vi "hcE_fortran.vi"(4 "nd":i32, 5 "ng":i32, 6 "ns":i32, 7 "n":i32, 9 "d":dbl[](array[numeric]), 10 "ic":i32[](array[numeric]), 11 "x (data)":dbl[](array[numeric])) -> (1 "d (out)":dbl[](array[numeric]), 2 "ic (out)":i32[](array[numeric]), 3 "x (data out)":dbl[](array[numeric]))   [LabVIEW 2014]
panel:
  out "iopt":i32
  out "jopt":i32
  out "iold":i32
  out "jold":i32
  out "dold":dbl
  out "dij":dbl
  out "jk":i32
  out "ik":i32
  out "ii":i32
  out "icj":i32
  out "ici":i32
  out "ij":i32
  out "dopt":dbl
  out "sij":dbl
  out "nj":i32
  out "rj":dbl
  out "sj":dbl
  out "si":dbl
  out "rij":dbl
  out "ri":dbl
  out "nij":i32
  out "ni":i32
  out "FLMAX":dbl=1.797693134862e+308
  out "k":i32
  out "m":i32
  out "j":i32
  out "i":i32
  out "Is":i32
  out "Io":i32
  out "II":i32
  out "Id":i32
  out "Ig":i32
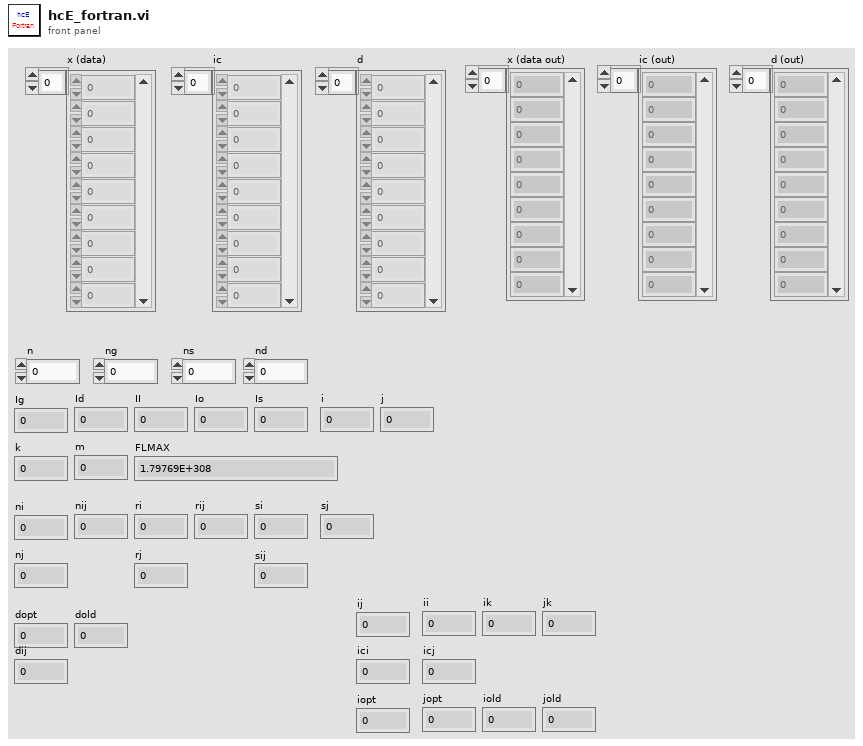
[diagram p1: front panel]
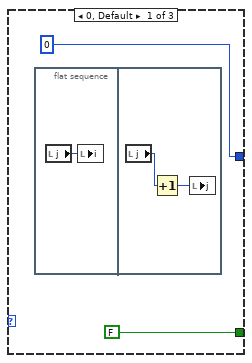
[diagram p2: hidden frame]
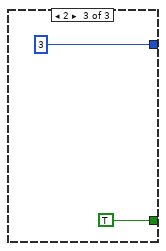
[diagram p3: hidden frame]
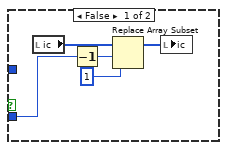
[diagram p6: hidden frame]
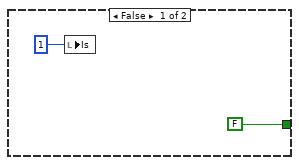
[diagram p8: hidden frame]
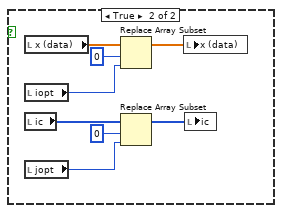
[diagram p9: hidden frame]
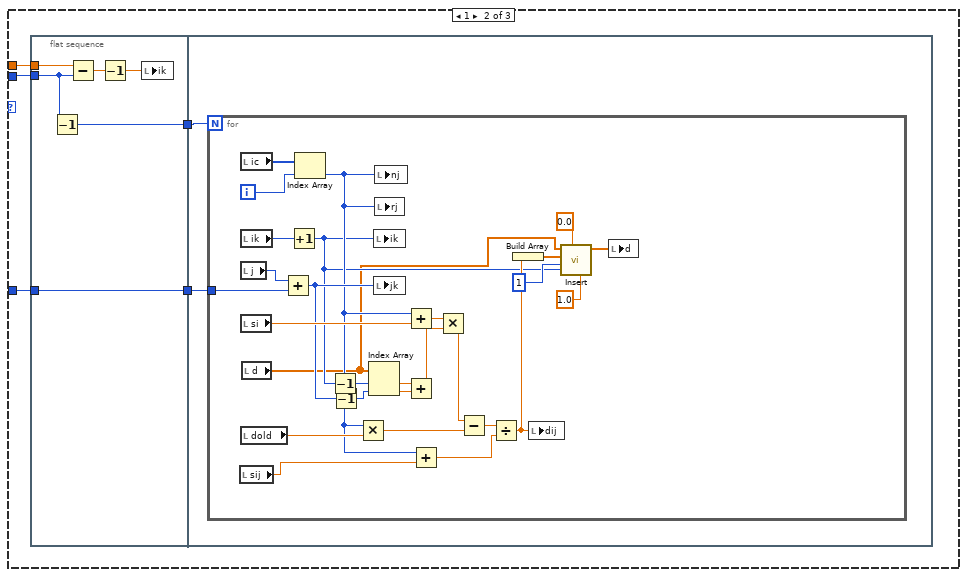
[diagram p12: hidden frame]
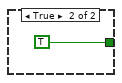
[diagram p13: hidden frame]
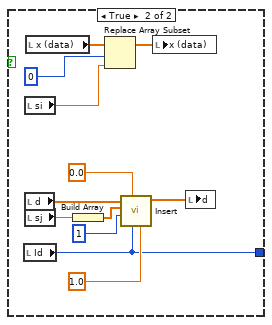
[diagram p14: hidden frame]
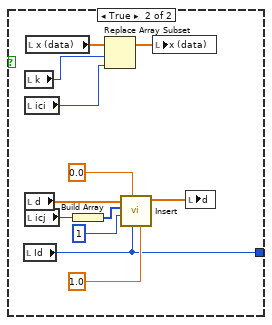
[diagram p16: hidden frame]
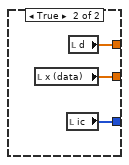
[diagram p17: hidden frame]
diagram:
  n1 = flat-sequence {
    tunnel: [w15] -> w5
    tunnel: w5 -> [w38]
    tunnel: [w37] -> w4
    tunnel: w4 -> [w188]
    tunnel: [w187] -> w2
    tunnel: [w186] -> w1
    tunnel: [w185] -> w3
    frame #0 {
      n2 = Decrement(x="ng") -> (x-1=w14:i32)
      n3 = Multiply(x="ng", y=w14) -> (x*y=w13:i32)
      n4 = Subtract(x="nd", y="ng") -> (x-y=→"II":i32)
      n5 = Divide(x=w13, y=2) -> (x/y=→"Id":dbl)
      "Ig" <- "ng"
      "Io" <- "nd"
      "i" <- 1 ("i")
      "j" <- 2 ("j")
    }
    frame #1 {
      # "i = 1\n      j = 2\n 1    continue\n        icj = ic(j)\n        if (icj .ne. j) goto 2\n        if (j .eq. lg)  goto 3\n        i = j\n        j = j + 1\n      goto 1"
      n6 = while {
        tunnel: [w17] -> w15
        i -> [w27]
        stop <- w18 stop-if-true
        # "j = 2\n(i or here is j)"
        n7 = local read "Ig"() -> (w23:i32)
        n8 = local read "ic"() -> (w26:i32[])
        n9 = Increment(x=w27) -> (x+1=w24:i32)
        n10 = Decrement(x=w24) -> (x-1=w16:i32)
        n11 = Index Array(array=w26, index=w16) -> (element=w25:i32)
        n12 = Equal?(x=w23, y=w24) -> (x = y?=w21:bool)
        n13 = Not Equal?(x=w24, y=w25) -> (x != y?=w22:bool)
        n14 = Build Array(w22, w21) -> (w20:bool[])
        n15 = call "Case_Selector.vi"("Array"=w20) -> ("Case Numer"=w19:i32)  [unwired: 10 in]
        n16 = case shown="1" w19 {
          tunnel: [FALSE TRUE TRUE] -> w18
          tunnel: [0 2 3] -> w17
          frame 0, Default {
            n17 = flat-sequence {
              frame #0 {
                n18 = local read "j"() -> (w30:i32)
                n19 = local write "i"(w30) -> ()
              }
              frame #1 {
                n20 = local read "j"() -> (w32:i32)
                n21 = Increment(x=w32) -> (x+1=w31:i32)
                n22 = local write "j"(w31) -> ()
              }
            }
          }
          frame 1 {
          }
          frame 2 {
          }
        }
      }
    }
    frame #2 {
      # "Fortran statement 2 and 3 part"
      n23 = flat-sequence {
        tunnel: w38 -> [w39]
        tunnel: [w68] -> w37
        frame #0 {
          # "Fortran statement 2"
          n24 = case shown="2, Default" w39 {
            frame 2, Default {
              n25 = flat-sequence {
                frame #0 {
                  n26 = local read "i"() -> (w42:i32)
                  n27 = local read "j"() -> (w40:i32)
                  n28 = Increment(x=w40) -> (x+1=w41:i32)
                  n29 = local write "k"(w42) -> ()
                  n30 = local write "m"(w41) -> ()
                }
                frame #1 {
                  n31 = while {
                    i -> [w52]
                    stop <- w49 stop-if-true
                    n32 = local read "ic"() -> (w47:i32[])
                    n33 = local read "k"() -> (w46:i32)
                    n34 = local read "m"() -> (w51:i32)
                    n35 = local read "n"() -> (w50:i32)
                    n36 = Add(x=w51, y=w52) -> (x+y=w48:i32)
                    n37 = Decrement(x=w48) -> (x-1=w44:i32)
                    n38 = Greater Or Equal?(x=w48, y=w50) -> (x >= y?=w49:bool)
                    n39 = local write "j"(w48) -> ()
                    n40 = Index Array(array=w47, index=w44) -> (element=w43:i32)
                    n41 = Greater?(x=w43, y=w46) -> (0:w45:bool)
                    n42 = case shown="True" w45 {
                      tunnel: w43 -> [_ w53]
                      frame False {
                      }
                      frame True {
                        n43 = flat-sequence {
                          tunnel: [w55] -> w54
                          tunnel: w53 -> [w55]
                          tunnel: w54 -> [w61]
                          frame #0 {
                            n44 = local read "k"() -> (w57:i32)
                            n45 = Increment(x=w57) -> (x+1=w56:i32)
                            n46 = local write "k"(w56) -> ()
                          }
                          frame #1 {
                            n47 = local read "x (data)"() -> (w67:dbl[])
                            n48 = local read "k"() -> (w64:i32)
                            n49 = local read "j"() -> (w63:i32)
                            n50 = local read "ic"() -> (w65:i32[])
                            n51 = Decrement(x=w64) -> (x-1=w60:i32)
                            n52 = call "swap.vi"("j"=w63, "k"=w64, "Array"=w67) -> ("Array (swap)"=w66:dbl[])  [unwired: 8 in]
                            n53 = Index Array(array=w65, index=w60) -> (element=w62:i32)
                            n54 = Decrement(x=w63) -> (x-1=w59:i32)
                            n55 = Replace Array Subset(array=w65, new element #1=w62, index #1=w59, new element #2=w61, index #2=w60) -> (w58:i32[])
                            n56 = local write "x (data)"(w66) -> ()
                            n57 = local write "ic"(w58) -> ()
                          }
                        }
                      }
                    }
                  }
                }
              }
            }
            frame 3 {
            }
          }
        }
        frame #1 {
          # "Fortran statement 3"
          n58 = flat-sequence {
            tunnel: [w156] -> w68
            frame #0 {
              n59 = while {
                i -> [w72]
                stop <- w74 stop-if-true
                n60 = local read "ic"() -> (w73:i32[])
                n61 = local read "n"() -> (w75:i32)
                n62 = Increment(x=w72) -> (x+1=w70:i32)
                n63 = Index Array(array=w73, index=w72) -> (element=w69:i32)
                n64 = Greater Or Equal?(x=w70, y=w75) -> (x >= y?=w74:bool)
                n65 = local write "i"(w69) -> ()
                n66 = local write "j"(w70) -> ()
                n67 = Not Equal?(x=w69, y=w70) -> (x != y?=w71:bool)
                n68 = case shown="True" w71 {
                  tunnel: w70 -> [w79 w82]
                  tunnel: w69 -> [_ w81]
                  frame False {
                    n69 = local read "ic"() -> (w80:i32[])
                    n70 = Decrement(x=w79) -> (x-1=w78:i32)
                    n71 = Replace Array Subset(array=w80, new element=1 ("new element/subarray"), index=w78) -> (w76:i32[])
                    n72 = local write "ic"(w76) -> ()
                  }
                  frame True {
                    n73 = flat-sequence {
                      tunnel: w82 -> [w91]
                      tunnel: w81 -> [w87]
                      frame #0 {
                        n74 = Decrement(x=w87) -> (x-1=w85:i32)
                        n75 = local read "ic"() -> (w88:i32[])
                        n76 = Decrement(x=w91) -> (x-1=w90:i32)
                        n77 = Index Array(array=w88, index=w85) -> (element=w86:i32)
                        n78 = Increment(x=w86) -> (x+1=w84:i32)
                        n79 = local write "nij"(w84) -> ()
                        n80 = local write "ni"(w86) -> ()
                        n81 = Replace Array Subset(array=w88, new element #1=0 ("new element/subarray"), index #1=w90, new element #2=w84, index #2=w85) -> (w83:i32[])
                        n82 = local write "ic"(w83) -> ()
                      }
                      frame #1 {
                        n83 = local read "nij"() -> (w107:i32)
                        n84 = local read "ni"() -> (w105:i32)
                        n85 = local read "x (data)"() -> (w96:dbl[])
                        n86 = local read "i"() -> (w104:i32)
                        n87 = local read "j"() -> (w103:i32)
                        n88 = Decrement(x=w103) -> (x-1=w95:i32)
                        n89 = Decrement(x=w104) -> (x-1=w94:i32)
                        n90 = Divide(x=1.0, y=w107) -> (x/y=w106:dbl)
                        n91 = Index Array(array=w96, index #1=w94, index #2=w95) -> (element #1=w102:dbl, element #2=w101:dbl)
                        n92 = Square Root(x=w106) -> (sqrt(x)=w99:dbl)
                        n93 = Multiply(x=w99, y=w105) -> (x*y=w100:dbl)
                        n94 = Multiply(x=w102, y=w100) -> (x*y=w98:dbl)
                        n95 = Multiply(x=w101, y=w99) -> (x*y=w97:dbl)
                        n96 = local write "rij"(w107) -> ()
                        n97 = local write "sj"(w99) -> ()
                        n98 = local write "si"(w100) -> ()
                        n99 = local write "ri"(w105) -> ()
                        n100 = Add(x=w98, y=w97) -> (x+y=w93:dbl)
                        n101 = Replace Array Subset(array=w96, new element=w93, index=w94) -> (w92:dbl[])
                        n102 = local write "x (data)"(w92) -> ()
                      }
                    }
                  }
                }
              }
            }
            frame #1 {
              n103 = local read "FLMAX"() -> (w110:dbl)
              n104 = local write "dopt"(w110) -> ()
              n105 = local write "ij"(0 ("ij")) -> ()
            }
            frame #2 {
              n106 = while {
                i -> [w115]
                stop <- w112 stop-if-true
                n107 = local read "Ig"() -> (w113:i32)
                n108 = flat-sequence {
                  tunnel: w111 -> [w119]
                  frame #0 {
                    n109 = local read "ic"() -> (w118:i32[])
                    n110 = Decrement(x=w119) -> (x-1=w117:i32)
                    n111 = local write "j"(w119) -> ()
                    n112 = Index Array(array=w118, index=w117) -> (element=w116:i32)
                    n113 = local write "rij"(w116) -> ()
                    n114 = local write "nj"(w116) -> ()
                  }
                  frame #1 {
                    n115 = while {
                      i -> [w141]
                      stop <- w150 stop-if-true
                      # "x(i), x(j)"
                      # "ic(i)"
                      n116 = local read "ic"() -> (w149:i32[])
                      n117 = local read "j"() -> (w152:i32)
                      n118 = Increment(x=w141) -> (x+1=w120:i32)
                      n119 = Decrement(x=w152) -> (x-1=w151:i32)
                      n120 = Index Array(array=w149, index=w141) -> (element=w147:i32)
                      n121 = local read "nj"() -> (w148:i32)
                      n122 = local read "rij"() -> (w143:dbl)
                      n123 = local read "x (data)"() -> (w142:dbl[])
                      n124 = local read "j"() -> (w140:i32)
                      n125 = local read "dopt"() -> (w122:dbl)
                      n126 = local read "d"() -> (w129:dbl[])
                      n127 = local read "ij"() -> (w131:i32)
                      n128 = Greater Or Equal?(x=w120, y=w151) -> (x >= y?=w150:bool)
                      n129 = Decrement(x=w140) -> (x-1=w139:i32)
                      n130 = Increment(x=w131) -> (x+1=w126:i32)
                      n131 = local write "i"(w120) -> ()
                      n132 = Add(x=w147, y=w148) -> (x+y=w144:i32)
                      n133 = Divide(x=w147, y=w144) -> (x/y=w145:dbl)
                      n134 = Divide(x=w143, y=w144) -> (x/y=w146:dbl)
                      n135 = Index Array(array=w142, index #1=w141, index #2=w139) -> (element #1=w138:dbl, element #2=w136:dbl)
                      n136 = Square Root(x=w145) -> (sqrt(x)=w135:dbl)
                      n137 = Square Root(x=w146) -> (sqrt(x)=w137:dbl)
                      n138 = Multiply(x=w138, y=w137) -> (x*y=w134:dbl)
                      n139 = Multiply(x=w136, y=w135) -> (x*y=w133:dbl)
                      n140 = Subtract(x=w134, y=w133) -> (x-y=w132:dbl)
                      n141 = Square(x=w132) -> (x^2=w121:dbl)
                      n142 = Less Or Equal?(x=w121, y=w122) -> (x <= y?=w123:bool)
                      n143 = case shown="True" w123 {
                        tunnel: w121 -> [_ w155]
                        tunnel: w120 -> [_ w154]
                        frame False {
                        }
                        frame True {
                          n144 = local read "j"() -> (w153:i32)
                          n145 = local write "dopt"(w155) -> ()
                          n146 = local write "iopt"(w154) -> ()
                          n147 = local write "jopt"(w153) -> ()
                        }
                      }
                      n148 = Build Array(w121) -> (w124:dbl[])
                      n149 = call "Insert.vi"("da"=1.0, "iy"=w126, "dy weight"=0.0, "ix"=1 ("iy"), "dx"=w124, "dy in"=w129) -> ("dy out"=w128:dbl[])  [unwired: 5 in]
                      n150 = local write "dij"(w121) -> ()
                      n151 = local write "ni"(w147) -> ()
                      n152 = local write "ri"(w147) -> ()
                      n153 = local write "nij"(w144) -> ()
                      n154 = local write "rij"(w144) -> ()
                      n155 = local write "si"(w135) -> ()
                      n156 = local write "sj"(w137) -> ()
                      n157 = local write "d"(w128) -> ()
                      n158 = local write "ij"(w126) -> ()
                    }
                  }
                }
                n159 = Add(x=w115, y=2) -> (x+y=w111:i32)
                n160 = Greater Or Equal?(x=w111, y=w113) -> (x >= y?=w112:bool)
              }
            }
            frame #3 {
              n161 = local read "ns"() -> (w159:i32)
              n162 = Equal?(x=w159, y=1) -> (x = y?=w157:bool)
              n163 = case shown="True" w157 {
                tunnel: [FALSE TRUE] -> w156
                frame False {
                  n164 = local write "Is"(1 ("Is")) -> ()
                }
                frame True {
                  n165 = local read "d"() -> (w167:dbl[])
                  n166 = local read "iopt"() -> (w164:i32)
                  n167 = local read "jopt"() -> (w163:i32)
                  n168 = Less?(x=w164, y=w163) -> (x < y?=w162:bool)
                  n169 = Index Array(array=w167, index=0) -> (element=w165:dbl)
                  n170 = case shown="False" w162 {
                    frame False {
                      n171 = local read "x (data)"() -> (w176:dbl[])
                      n172 = local read "jopt"() -> (w174:i32)
                      n173 = local read "ic"() -> (w170:i32[])
                      n174 = local read "iopt"() -> (w172:i32)
                      n175 = Replace Array Subset(array=w176, new element=w174, index=0) -> (w173:dbl[])
                      n176 = Replace Array Subset(array=w170, new element=w172, index=0) -> (w169:i32[])
                      n177 = local write "x (data)"(w173) -> ()
                      n178 = local write "ic"(w169) -> ()
                    }
                    frame True {
                      n179 = local read "x (data)"() -> (w184:dbl[])
                      n180 = local read "iopt"() -> (w182:i32)
                      n181 = local read "ic"() -> (w178:i32[])
                      n182 = local read "jopt"() -> (w180:i32)
                      n183 = Replace Array Subset(array=w184, new element=w182, index=0) -> (w181:dbl[])
                      n184 = Replace Array Subset(array=w178, new element=w180, index=0) -> (w177:i32[])
                      n185 = local write "x (data)"(w181) -> ()
                      n186 = local write "ic"(w177) -> ()
                    }
                  }
                  n187 = local write "dopt"(w165) -> ()
                }
              }
            }
          }
        }
      }
    }
    frame #3 {
      # "Fortran statement 100 and 300 part\nif ns == 1 than it should pass this part and return \n\n ****************************************************\n\n<prior parts...>\nif (ns .eq. 1) then\n        if (iopt .lt. jopt) then\n          x(1)  = dble(iopt)\n          ic(1) = jopt\n        else\n          x(1)  = dble(jopt)\n          ic(1) = iopt\n        end if\n        d(1)    = dopt\n        return\n      end if"
      n188 = case shown="False" w188 {
        tunnel: [w191 w527] -> w187
        tunnel: [w189 w526] -> w186
        tunnel: [w190 w525] -> w185
        frame False {
          n189 = flat-sequence {
            tunnel: [w351] -> w191
            tunnel: [w350] -> w190
            tunnel: [w349] -> w189
            frame #0 {
              # "Fortran statement 100"
              n190 = while {
                stop <- w192 stop-if-true
                n191 = flat-sequence {
                  tunnel: [w342] -> w192
                  frame #0 {
                    n192 = local read "ic"() -> (w200:i32[])
                    n193 = local read "iopt"() -> (w196:i32)
                    n194 = local read "jopt"() -> (w193:i32)
                    n195 = Decrement(x=w196) -> (x-1=w197:i32)
                    n196 = Decrement(x=w193) -> (x-1=w198:i32)
                    n197 = Index Array(array=w200, index #1=w197, index #2=w198) -> (element #1=w202:i32, element #2=w201:i32)
                    n198 = Add(x=w202, y=w201) -> (x+y=w199:i32)
                    n199 = Negate(x=w196) -> (-x=w195:i32)
                    n200 = Replace Array Subset(array=w200, new element #1=w199, index #1=w197, new element #2=w195, index #2=w198) -> (w194:i32[])
                    n201 = local write "ni"(w202) -> ()
                    n202 = local write "nj"(w201) -> ()
                    n203 = local write "nij"(w199) -> ()
                    n204 = local write "ic"(w194) -> ()
                  }
                  frame #1 {
                    n205 = local read "jopt"() -> (w209:i32)
                    n206 = local read "Ig"() -> (w210:i32)
                    n207 = local read "ni"() -> (w208:i32)
                    n208 = local read "nj"() -> (w207:i32)
                    n209 = local read "nij"() -> (w206:i32)
                    n210 = local read "dopt"() -> (w205:dbl)
                    n211 = local read "iopt"() -> (w204:i32)
                    n212 = local read "jopt"() -> (w203:i32)
                    n213 = Not Equal?(x=w209, y=w210) -> (x != y?=w211:bool)
                    n214 = case shown="True" w211 {
                      frame False {
                      }
                      frame True {
                        n215 = local read "ic"() -> (w215:i32[])
                        n216 = local read "d"() -> (w217:dbl[])
                        n217 = local read "jopt"() -> (w213:i32)
                        n218 = local read "Ig"() -> (w212:i32)
                        n219 = call "swap.vi"("j"=w212, "k"=w213, "Array"=w215) -> ("Array (swap)"=w214:dbl[])  [unwired: 8 in]
                        n220 = call "wardsw.vi"("n"=w212, "i"=w213, "d"=w217) -> ("d(wardsw)"=w216:dbl[])  [unwired: 8 in]
                        n221 = local write "ic"(w214) -> ()
                        n222 = local write "d"(w216) -> ()
                      }
                    }
                    n223 = local write "si"(w208) -> ()
                    n224 = local write "sj"(w207) -> ()
                    n225 = local write "sij"(w206) -> ()
                    n226 = local write "dold"(w205) -> ()
                    n227 = local write "iold"(w204) -> ()
                    n228 = local write "jold"(w203) -> ()
                  }
                  frame #2 {
                    w233 = -1 ("jopt")
                    n229 = local read "FLMAX"() -> (w232:dbl)
                    n230 = local read "Ig"() -> (w231:i32)
                    n231 = local read "Id"() -> (w230:i32)
                    n232 = local read "iold"() -> (w219:i32)
                    n233 = Decrement(x=w231) -> (x-1=w225:i32)
                    n234 = Decrement(x=w219) -> (x-1=w229:i32)
                    n235 = Multiply(x=w219, y=w229) -> (x*y=w228:i32)
                    n236 = Divide(x=w228, y=2) -> (x/y=w220:dbl)
                    n237 = local write "ii"(w220) -> ()
                    n238 = Greater?(x=w219, y=1) -> (0:w224:bool)
                    n239 = Less?(x=w219, y=w225) -> (x < y?=w223:bool)
                    n240 = Subtract(x=w230, y=w225) -> (x-y=w218:i32)
                    n241 = Build Array(w224, w223) -> (w221:bool[])
                    n242 = call "Case_Selector.vi"("Array"=w221) -> ("Case Numer"=w222:i32)  [unwired: 10 in]
                    n243 = local write "jopt"(w233) -> ()
                    n244 = local write "iopt"(w233) -> ()
                    n245 = local write "dopt"(w232) -> ()
                    n246 = local write "Ig"(w225) -> ()
                    n247 = local write "Id"(w218) -> ()
                    n248 = case shown="2" w222 {
                      tunnel: w220 -> [_ w238 w279]
                      tunnel: w219 -> [_ w237 w278]
                      tunnel: w218 -> [_ w235 w277]
                      frame 0, Default {
                      }
                      frame 1 {
                        n249 = flat-sequence {
                          tunnel: w238 -> [w244]
                          tunnel: w237 -> [w241]
                          tunnel: [w240] -> w236
                          tunnel: w235 -> [w239]
                          tunnel: [w239] -> w234
                          tunnel: w236 -> [w246]
                          tunnel: w234 -> [w245]
                          frame #0 {
                            n250 = Decrement(x=w241) -> (x-1=w240:i32)
                            n251 = Subtract(x=w244, y=w241) -> (x-y=w243:dbl)
                            n252 = Decrement(x=w243) -> (x-1=w242:dbl)
                            n253 = local write "ik"(w242) -> ()
                          }
                          frame #1 {
                            n254 = for {
                              N: w246 -> [_]
                              tunnel: w245 -> [w270]
                              i -> [w273]
                              n255 = local read "sij"() -> (w256:dbl)
                              n256 = local read "ic"() -> (w274:i32[])
                              n257 = local read "ik"() -> (w272:i32)
                              n258 = local read "j"() -> (w271:i32)
                              n259 = local read "si"() -> (w269:dbl)
                              n260 = local read "dold"() -> (w260:dbl)
                              n261 = local read "d"() -> (w247:dbl[])
                              n262 = Add(x=w271, y=w270) -> (x+y=w266:i32)
                              n263 = Increment(x=w272) -> (x+1=w249:i32)
                              n264 = Index Array(array=w274, index=w273) -> (element=w257:i32)
                              n265 = Decrement(x=w249) -> (x-1=w268:i32)
                              n266 = Decrement(x=w266) -> (x-1=w267:i32)
                              n267 = Multiply(x=w257, y=w260) -> (x*y=w259:dbl)
                              n268 = Index Array(array=w247, index #1=w268, index #2=w267) -> (element #1=w265:dbl, element #2=w264:dbl)
                              n269 = local write "ik"(w249) -> ()
                              n270 = local write "jk"(w266) -> ()
                              n271 = local write "nj"(w257) -> ()
                              n272 = local write "rj"(w257) -> ()
                              n273 = Add(x=w257, y=w269) -> (x+y=w263:dbl)
                              n274 = Add(x=w265, y=w264) -> (x+y=w262:dbl)
                              n275 = Add(x=w257, y=w256) -> (x+y=w255:dbl)
                              n276 = Multiply(x=w263, y=w262) -> (x*y=w261:dbl)
                              n277 = Subtract(x=w261, y=w259) -> (x-y=w258:dbl)
                              n278 = Divide(x=w258, y=w255) -> (x/y=w253:dbl)
                              n279 = Build Array(w253) -> (w254:dbl[])
                              n280 = local write "dij"(w253) -> ()
                              n281 = call "Insert.vi"("da"=1.0, "iy"=w249, "dy weight"=0.0, "ix"=1, "dx"=w254, "dy in"=w247) -> ("dy out"=w248:dbl[])  [unwired: 5 in]
                              n282 = local write "d"(w248) -> ()
                            }
                          }
                        }
                      }
                      frame 2 {
                        n283 = flat-sequence {
                          tunnel: w279 -> [w285]
                          tunnel: w278 -> [w284]
                          tunnel: w277 -> [w283]
                          tunnel: [w283] -> w276
                          tunnel: [w280] -> w275
                          tunnel: w276 -> [w287]
                          tunnel: w275 -> [w286]
                          frame #0 {
                            n284 = local read "iold"() -> (w281:i32)
                            n285 = Add(x=w285, y=w284) -> (x+y=w282:dbl)
                            n286 = Increment(x=w281) -> (x+1=w280:i32)
                            n287 = local write "ik"(w282) -> ()
                            n288 = local write "i"(w281) -> ()
                          }
                          frame #1 {
                            n289 = for {
                              N: w286 -> [_]
                              tunnel: w287 -> [w288]
                              i -> [w289]
                              n290 = flat-sequence {
                                tunnel: w289 -> [w315]
                                tunnel: w288 -> [w313]
                                frame #0 {
                                n291 = local read "sij"() -> (w299:dbl)
                                n292 = local read "ic"() -> (w316:i32[])
                                n293 = local read "j"() -> (w314:i32)
                                n294 = local read "si"() -> (w312:dbl)
                                n295 = local read "ik"() -> (w290:i32)
                                n296 = local read "dold"() -> (w303:dbl)
                                n297 = local read "d"() -> (w291:dbl[])
                                n298 = Add(x=w314, y=w313) -> (x+y=w309:i32)
                                n299 = Index Array(array=w316, index=w315) -> (element=w300:i32)
                                n300 = Decrement(x=w290) -> (x-1=w311:i32)
                                n301 = Decrement(x=w309) -> (x-1=w310:i32)
                                n302 = Multiply(x=w300, y=w303) -> (x*y=w302:dbl)
                                n303 = Index Array(array=w291, index #1=w311, index #2=w310) -> (element #1=w308:dbl, element #2=w307:dbl)
                                n304 = local write "jk"(w309) -> ()
                                n305 = local write "nj"(w300) -> ()
                                n306 = local write "rj"(w300) -> ()
                                n307 = Add(x=w300, y=w312) -> (x+y=w306:dbl)
                                n308 = Add(x=w308, y=w307) -> (x+y=w305:dbl)
                                n309 = Add(x=w300, y=w299) -> (x+y=w298:dbl)
                                n310 = Multiply(x=w306, y=w305) -> (x*y=w304:dbl)
                                n311 = Subtract(x=w304, y=w302) -> (x-y=w301:dbl)
                                n312 = Divide(x=w301, y=w298) -> (x/y=w296:dbl)
                                n313 = Build Array(w296) -> (w297:dbl[])
                                n314 = local write "dij"(w296) -> ()
                                n315 = call "Insert.vi"("da"=1.0, "iy"=w290, "dy weight"=0.0, "ix"=1, "dx"=w297, "dy in"=w291) -> ("dy out"=w292:dbl[])  [unwired: 5 in]
                                n316 = local write "d"(w292) -> ()
                                }
                                frame #1 {
                                n317 = local read "ik"() -> (w319:i32)
                                n318 = local read "i"() -> (w318:i32)
                                n319 = Add(x=w319, y=w318) -> (x+y=w317:i32)
                                n320 = local write "ik"(w317) -> ()
                                }
                                frame #2 {
                                n321 = local read "j"() -> (w320:i32)
                                n322 = local write "i"(w320) -> ()
                                }
                              }
                            }
                          }
                        }
                      }
                    }
                  }
                  frame #3 {
                    w332 = 1
                    w333 = 0.0 ("dy weight")
                    w341 = 1.0 ("da")
                    n323 = local read "dold"() -> (w331:dbl)
                    n324 = local read "iold"() -> (w330:i32)
                    n325 = local read "jold"() -> (w329:i32)
                    n326 = local read "d"() -> (w336:dbl[])
                    n327 = local read "Io"() -> (w338:i32)
                    n328 = local write "jopt"(2) -> ()
                    n329 = local write "iopt"(1) -> ()
                    n330 = Build Array(w331) -> (w328:dbl[])
                    n331 = Build Array(w330) -> (w327:i32[])
                    n332 = Build Array(w329) -> (w326:i32[])
                    n333 = call "Insert.vi"("da"=w341, "iy"=w338, "dy weight"=w333, "ix"=w332, "dx"=w328, "dy in"=w336) -> ("dy out"=w335:dbl[])  [unwired: 5 in]
                    n334 = Decrement(x=w338) -> (x-1=w340:i32)
                    n335 = Subtract(x=w338, y=2) -> (x-y=w339:i32)
                    n336 = call "Insert.vi"("da"=w341, "iy"=w340, "dy weight"=w333, "ix"=w332, "dx"=w327, "dy in"=w335) -> ("dy out"=w334:dbl[])  [unwired: 5 in]
                    n337 = call "Insert.vi"("da"=w341, "iy"=w339, "dy weight"=w333, "ix"=w332, "dx"=w326, "dy in"=w334) -> ("dy out"=w323:dbl[])  [unwired: 5 in]
                    n338 = Index Array(array=w323, index=0) -> (element=w321:dbl)
                    n339 = local write "d"(w323) -> ()
                    n340 = local write "dopt"(w321) -> ()
                  }
                  frame #4 {
                    n341 = local read "Is"() -> (w346:i32)
                    n342 = local read "ns"() -> (w343:i32)
                    n343 = Increment(x=w346) -> (x+1=w344:i32)
                    n344 = Equal?(x=w344, y=w343) -> (x = y?=w345:bool)
                    n345 = case shown="False" w345 {
                      tunnel: [FALSE TRUE] -> w342
                      frame False {
                      }
                      frame True {
                      }
                    }
                    n346 = local write "Is"(w344) -> ()
                  }
                }
              }
            }
            frame #1 {
              # "Fortran statement 900"
              n347 = flat-sequence {
                tunnel: [w524] -> w351
                tunnel: [w523] -> w350
                tunnel: [w522] -> w349
                frame #0 {
                  w360 = 1
                  w361 = 0.0 ("dy weight")
                  w369 = 1.0 ("da")
                  n348 = local read "dold"() -> (w359:dbl)
                  n349 = local read "iold"() -> (w358:i32)
                  n350 = local read "jold"() -> (w357:i32)
                  n351 = local read "d"() -> (w364:dbl[])
                  n352 = local read "Io"() -> (w366:i32)
                  n353 = local read "ng"() -> (w352:i32)
                  n354 = Build Array(w359) -> (w356:dbl[])
                  n355 = Build Array(w358) -> (w355:i32[])
                  n356 = Build Array(w357) -> (w354:i32[])
                  n357 = for {
                    N: w352 -> [_]
                    i -> [w372]
                    n358 = local read "ic"() -> (w373:i32[])
                    n359 = Increment(x=w372) -> (x+1=w371:i32)
                    n360 = Replace Array Subset(array=w373, new element=w371, index=w372) -> (w370:i32[])
                    n361 = local write "ic"(w370) -> ()
                  }
                  n362 = call "Insert.vi"("da"=w369, "iy"=w366, "dy weight"=w361, "ix"=w360, "dx"=w356, "dy in"=w364) -> ("dy out"=w363:dbl[])  [unwired: 5 in]
                  n363 = Decrement(x=w366) -> (x-1=w368:i32)
                  n364 = Subtract(x=w366, y=2) -> (x-y=w367:i32)
                  n365 = call "Insert.vi"("da"=w369, "iy"=w368, "dy weight"=w361, "ix"=w360, "dx"=w355, "dy in"=w363) -> ("dy out"=w362:dbl[])  [unwired: 5 in]
                  n366 = call "Insert.vi"("da"=w369, "iy"=w367, "dy weight"=w361, "ix"=w360, "dx"=w354, "dy in"=w362) -> ("dy out"=w353:dbl[])  [unwired: 5 in]
                  n367 = local write "d"(w353) -> ()
                }
                frame #1 {
                  n368 = local read "nd"() -> (w385:i32)
                  n369 = local read "d"() -> (w384:dbl[])
                  n370 = local read "ic"() -> (w378:i32[])
                  n371 = local read "ng"() -> (w377:i32)
                  n372 = Decrement(x=w385) -> (x-1=w383:i32)
                  n373 = Decrement(x=w383) -> (x-1=w375:i32)
                  n374 = Decrement(x=w383) -> (x-1=w382:i32)
                  n375 = Decrement(x=w382) -> (x-1=w374:i32)
                  n376 = Index Array(array=w384, index #1=w375, index #2=w374) -> (element #1=w381:dbl, element #2=w380:dbl)
                  n377 = To Long Integer(number=w380) -> (32bit integer=w379:i32)
                  n378 = local write "Io"(w382) -> ()
                  n379 = local write "Id"(w383) -> ()
                  n380 = local write "si"(w381) -> ()
                  n381 = local write "sj"(w380) -> ()
                  n382 = Replace Array Subset(array=w378, new element=w377, index=w379) -> (w376:i32[])
                  n383 = local write "ic"(w376) -> ()
                }
                frame #2 {
                  n384 = local read "si"() -> (w392:dbl)
                  n385 = local read "sj"() -> (w391:dbl)
                  n386 = local read "ng"() -> (w387:i32)
                  n387 = Less?(x=w392, y=w391) -> (x < y?=w390:bool)
                  n388 = case shown="False" w390 {
                    tunnel: [w393 w405] -> w389
                    frame False {
                      n389 = local read "Id"() -> (w393:i32)
                      n390 = local read "sj"() -> (w401:dbl)
                      n391 = local read "d"() -> (w395:dbl[])
                      n392 = local read "si"() -> (w398:dbl)
                      n393 = local read "x (data)"() -> (w404:dbl[])
                      n394 = Build Array(w398) -> (w397:dbl[])
                      n395 = Replace Array Subset(array=w404, new element=w401, index=0) -> (w402:dbl[])
                      n396 = call "Insert.vi"("da"=1.0, "iy"=w393, "dy weight"=0.0, "ix"=1, "dx"=w397, "dy in"=w395) -> ("dy out"=w394:dbl[])  [unwired: 5 in]
                      n397 = local write "x (data)"(w402) -> ()
                      n398 = local write "d"(w394) -> ()
                    }
                    frame True {
                      n399 = local read "Id"() -> (w405:i32)
                      n400 = local read "si"() -> (w413:dbl)
                      n401 = local read "d"() -> (w407:dbl[])
                      n402 = local read "sj"() -> (w410:dbl)
                      n403 = local read "x (data)"() -> (w416:dbl[])
                      n404 = Build Array(w410) -> (w409:dbl[])
                      n405 = Replace Array Subset(array=w416, new element=w413, index=0) -> (w414:dbl[])
                      n406 = call "Insert.vi"("da"=1.0, "iy"=w405, "dy weight"=0.0, "ix"=1, "dx"=w409, "dy in"=w407) -> ("dy out"=w406:dbl[])  [unwired: 5 in]
                      n407 = local write "x (data)"(w414) -> ()
                      n408 = local write "d"(w406) -> ()
                    }
                  }
                  n409 = Decrement(x=w389) -> (x-1=w388:i32)
                  n410 = Increment(x=w387) -> (x+1=w386:i32)
                  n411 = local write "Id"(w388) -> ()
                  n412 = local write "Ig"(w386) -> ()
                }
                frame #3 {
                  n413 = while {
                    i -> [w421]
                    stop <- w417 stop-if-true
                    n414 = local read "ns"() -> (w418:i32)
                    n415 = flat-sequence {
                      frame #0 {
                        n416 = local read "d"() -> (w426:dbl[])
                        n417 = local read "Id"() -> (w423:i32)
                        n418 = local read "Io"() -> (w429:i32)
                        n419 = Decrement(x=w429) -> (x-1=w425:i32)
                        n420 = Decrement(x=w425) -> (x-1=w424:i32)
                        n421 = Decrement(x=w423) -> (x-1=w422:i32)
                        n422 = Index Array(array=w426, index=w424) -> (element=w427:dbl)
                        n423 = Replace Array Subset(array=w426, new element=w427, index=w422) -> (w428:dbl[])
                        n424 = local write "Id"(w422) -> ()
                        n425 = local write "Io"(w425) -> ()
                        n426 = local write "d"(w428) -> ()
                      }
                      frame #1 {
                        n427 = local read "d"() -> (w436:dbl[])
                        n428 = local read "Io"() -> (w435:i32)
                        n429 = Decrement(x=w435) -> (x-1=w437:i32)
                        n430 = Decrement(x=w437) -> (x-1=w438:i32)
                        n431 = Index Array(array=w436, index=w438) -> (element=w434:dbl)
                        n432 = To Long Integer(number=w434) -> (32bit integer=w433:i32)
                        n433 = local read "ic"() -> (w432:i32[])
                        n434 = Decrement(x=w433) -> (x-1=w430:i32)
                        n435 = local write "i"(w433) -> ()
                        n436 = local write "Io"(w437) -> ()
                        n437 = Index Array(array=w432, index=w430) -> (element=w431:i32)
                        n438 = local write "ici"(w431) -> ()
                      }
                      frame #2 {
                        n439 = local read "d"() -> (w441:dbl[])
                        n440 = local read "Io"() -> (w442:i32)
                        n441 = Decrement(x=w442) -> (x-1=w440:i32)
                        n442 = Decrement(x=w440) -> (x-1=w439:i32)
                        n443 = Index Array(array=w441, index=w439) -> (element=w443:dbl)
                        n444 = To Long Integer(number=w443) -> (32bit integer=w444:i32)
                        n445 = local read "ic"() -> (w445:i32[])
                        n446 = Decrement(x=w444) -> (x-1=w447:i32)
                        n447 = local write "j"(w444) -> ()
                        n448 = local write "Io"(w440) -> ()
                        n449 = Index Array(array=w445, index=w447) -> (element=w446:i32)
                        n450 = local write "icj"(w446) -> ()
                      }
                      frame #3 {
                        n451 = local read "ici"() -> (w460:i32)
                        n452 = local read "icj"() -> (w459:i32)
                        n453 = local read "ic"() -> (w455:i32[])
                        n454 = local read "j"() -> (w452:i32)
                        n455 = local read "ic"() -> (w454:i32[])
                        n456 = local read "Ig"() -> (w450:i32)
                        n457 = local read "k"() -> (w451:i32)
                        n458 = Decrement(x=w452) -> (x-1=w456:i32)
                        n459 = Greater?(x=w460, y=w459) -> (0:w458:bool)
                        n460 = Subtract(x=w450, y=w451) -> (x-y=w449:i32)
                        n461 = Decrement(x=w449) -> (x-1=w448:i32)
                        n462 = case shown="True" w458 {
                          frame False {
                          }
                          frame True {
                            n463 = local read "ic"() -> (w465:i32[])
                            n464 = local read "i"() -> (w463:i32)
                            n465 = local read "icj"() -> (w462:i32)
                            n466 = Decrement(x=w463) -> (x-1=w464:i32)
                            n467 = Replace Array Subset(array=w465, new element=w462, index=w464) -> (w461:i32[])
                            n468 = local write "ic"(w461) -> ()
                          }
                        }
                        n469 = Index Array(array=w454, index=w448) -> (element=w453:i32)
                        n470 = Replace Array Subset(array=w455, new element=w453, index=w456) -> (w457:i32[])
                        n471 = local write "ic"(w457) -> ()
                      }
                      frame #4 {
                        n472 = local read "ici"() -> (w470:i32)
                        n473 = local read "icj"() -> (w469:i32)
                        n474 = Less?(x=w470, y=w469) -> (x < y?=w468:bool)
                        n475 = case shown="False" w468 {
                          tunnel: [w472 w485] -> w467
                          frame False {
                            n476 = local read "ici"() -> (w477:i32)
                            n477 = local read "Id"() -> (w472:i32)
                            n478 = local read "d"() -> (w474:dbl[])
                            n479 = local read "x (data)"() -> (w482:dbl[])
                            n480 = local read "k"() -> (w471:i32)
                            n481 = local read "icj"() -> (w480:i32)
                            n482 = Build Array(w477) -> (w476:i32[])
                            n483 = Replace Array Subset(array=w482, new element=w480, index=w471) -> (w481:dbl[])
                            n484 = call "Insert.vi"("da"=1.0, "iy"=w472, "dy weight"=0.0, "ix"=1, "dx"=w476, "dy in"=w474) -> ("dy out"=w473:dbl[])  [unwired: 5 in]
                            n485 = local write "x (data)"(w481) -> ()
                            n486 = local write "d"(w473) -> ()
                          }
                          frame True {
                            n487 = local read "Id"() -> (w485:i32)
                            n488 = local read "k"() -> (w484:i32)
                            n489 = local read "ici"() -> (w483:i32)
                            n490 = local read "d"() -> (w487:dbl[])
                            n491 = local read "icj"() -> (w490:i32)
                            n492 = local read "x (data)"() -> (w494:dbl[])
                            n493 = Build Array(w490) -> (w489:i32[])
                            n494 = Replace Array Subset(array=w494, new element=w483, index=w484) -> (w493:dbl[])
                            n495 = call "Insert.vi"("da"=1.0, "iy"=w485, "dy weight"=0.0, "ix"=1, "dx"=w489, "dy in"=w487) -> ("dy out"=w486:dbl[])  [unwired: 5 in]
                            n496 = local write "x (data)"(w493) -> ()
                            n497 = local write "d"(w486) -> ()
                          }
                        }
                        n498 = Decrement(x=w467) -> (x-1=w466:i32)
                        n499 = local write "Id"(w466) -> ()
                      }
                    }
                    n500 = Add(x=w421, y=2) -> (x+y=w419:i32)
                    n501 = Greater Or Equal?(x=w419, y=w418) -> (x >= y?=w417:bool)
                  }
                }
                frame #4 {
                  n502 = local read "nd"() -> (w496:i32)
                  n503 = Decrement(x=w496) -> (x-1=w495:i32)
                  n504 = local write "Id"(w496) -> ()
                  n505 = local write "Io"(w495) -> ()
                }
                frame #5 {
                  n506 = local read "ns"() -> (w497:i32)
                  n507 = for {
                    N: w497 -> [_]
                    n508 = local read "ic"() -> (w512:i32[])
                    n509 = local read "k"() -> (w511:i32)
                    n510 = local read "d"() -> (w504:dbl[])
                    n511 = local read "Io"() -> (w510:i32)
                    n512 = local read "Id"() -> (w506:i32)
                    n513 = Decrement(x=w511) -> (x-1=w507:i32)
                    n514 = Decrement(x=w510) -> (x-1=w502:i32)
                    n515 = Decrement(x=w506) -> (x-1=w500:i32)
                    n516 = Index Array(array=w504, index=w502) -> (element=w509:dbl)
                    n517 = Decrement(x=w502) -> (x-1=w501:i32)
                    n518 = Decrement(x=w500) -> (x-1=w499:i32)
                    n519 = Replace Array Subset(array=w512, new element=w509, index=w507) -> (w508:i32[])
                    n520 = Decrement(x=w502) -> (x-1=w498:i32)
                    n521 = Index Array(array=w504, index=w501) -> (element=w505:dbl)
                    n522 = Replace Array Subset(array=w504, new element=w505, index=w499) -> (w503:dbl[])
                    n523 = local write "Io"(w498) -> ()
                    n524 = local write "Id"(w500) -> ()
                    n525 = local write "ic"(w508) -> ()
                    n526 = local write "d"(w503) -> ()
                  }
                }
                frame #6 {
                  n527 = local read "nd"() -> (w514:i32)
                  n528 = local write "Id"(w514) -> ()
                  n529 = local write "Io"(1 ("Io")) -> ()
                }
                frame #7 {
                  n530 = local read "ns"() -> (w515:i32)
                  n531 = for {
                    N: w515 -> [_]
                    n532 = local read "d"() -> (w521:dbl[])
                    n533 = local read "Io"() -> (w519:i32)
                    n534 = local read "Id"() -> (w518:i32)
                    n535 = call "swap.vi"("j"=w518, "k"=w519, "Array"=w521) -> ("Array (swap)"=w520:dbl[])  [unwired: 8 in]
                    n536 = Increment(x=w519) -> (x+1=w517:i32)
                    n537 = Decrement(x=w518) -> (x-1=w516:i32)
                    n538 = local write "Io"(w517) -> ()
                    n539 = local write "Id"(w516) -> ()
                    n540 = local write "d"(w520) -> ()
                  }
                }
                frame #8 {
                  n541 = local read "x (data)"() -> (w522:dbl[])
                  n542 = local read "ic"() -> (w523:i32[])
                  n543 = local read "d"() -> (w524:dbl[])
                }
              }
            }
          }
        }
        frame True {
          n544 = local read "x (data)"() -> (w526:dbl[])
          n545 = local read "ic"() -> (w525:i32[])
          n546 = local read "d"() -> (w527:dbl[])
        }
      }
    }
  }
  "ic (out)" <- w3
  "d (out)" <- w2
  "x (data out)" <- w1
